vi "POV To Buttons.vi"(11 "POV Value":i16) -> (0 "Button Released":T1, 1 "Button Pressed":T1, 3 "Buttons'  States":T1)   [LabVIEW 2014]
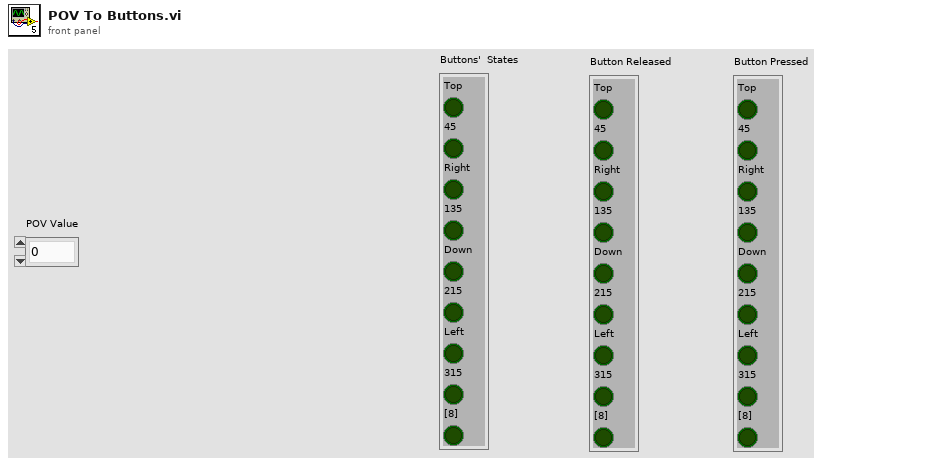
[diagram p1: front panel]
types:
  T1 = cluster{"Top":bool, "45":bool, "Right":bool, "135":bool, "Down":bool, "215":bool, "Left":bool, "315":bool, "[8]":bool}
  T2 = cluster{"[0]":bool, "[1]":bool, "[2]":bool, "[3]":bool, "[4]":bool, "[5]":bool, "[6]":bool, "[7]":bool, "[8]":bool}
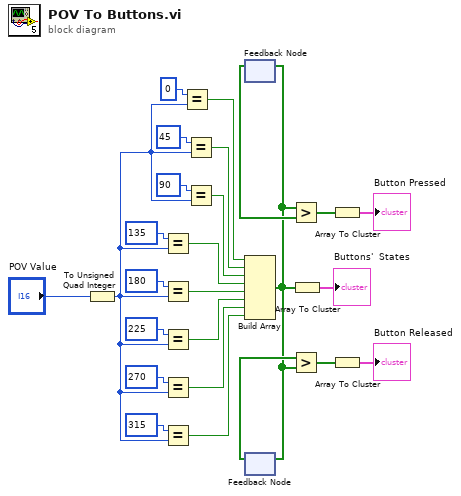
[diagram p0: block diagram]
diagram:
  n1 = To Unsigned Quad Integer(1:"POV Value") -> (0:w8:u64)
  n2 = Equal?(x=u64 135, y=w8) -> (x = y?=w20:bool)
  n3 = Equal?(x=u64 180, y=w8) -> (x = y?=w18:bool)
  n4 = Equal?(x=u64 225, y=w8) -> (x = y?=w16:bool)
  n5 = Equal?(x=u64 270, y=w8) -> (x = y?=w14:bool)
  n6 = Equal?(x=u64 315, y=w8) -> (x = y?=w12:bool)
  n7 = Equal?(x=u64 0, y=w8) -> (x = y?=w7:bool)
  n8 = Equal?(x=u64 45, y=w8) -> (x = y?=w24:bool)
  n9 = Equal?(x=u64 90, y=w8) -> (x = y?=w22:bool)
  n10 = feedback #1() -> (w9:bool[])  [unwired: 1 in]
  n11 = Build Array(w7, w24, w22, w20, w18, w16, w14, w12) -> (w1:bool[])
  n12 = feedback-in #1(w1) -> ()
  n13 = feedback #2() -> (w2:bool[])  [unwired: 1 in]
  n14 = feedback-in #2(w1) -> ()
  n15 = Greater?(x=w1, y=w9) -> (0:w5:bool[])
  n16 = Greater?(x=w2, y=w1) -> (0:w3:bool[])
  n17 = Array To Cluster(array=w1) -> (cluster=→"Buttons'  States":T2)
  n18 = Array To Cluster(array=w5) -> (cluster=→"Button Pressed":T2)
  n19 = Array To Cluster(array=w3) -> (cluster=→"Button Released":T2)
